vi "Package Must Exist.vi"(8 "error in (no error)":errorcluster, 11 "UpdateAction in":refnum<class "UpdateAction.lvclass">) -> (0 "error out":errorcluster, 2 "Pkg Must Exist":bool, 3 "UpdateAction out":refnum<class "UpdateAction.lvclass">)   [LabVIEW 2020, in "GPackTools.lvlib" / "UpdateAction.lvclass"]
uses:
  UpdateAction.lvclass
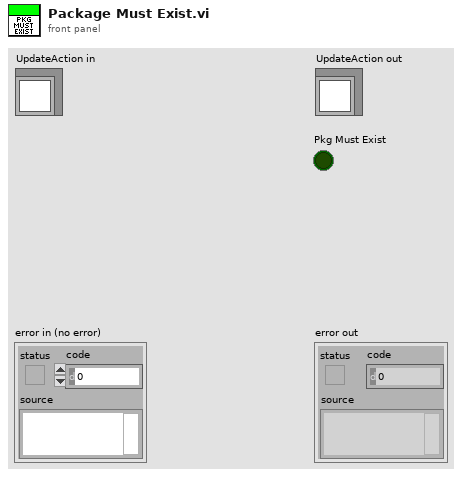
[diagram p1: front panel]
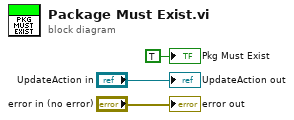
[diagram p0: block diagram]
diagram:
  "error out" <- "error in (no error)"
  "UpdateAction out" <- "UpdateAction in"
  "Pkg Must Exist" <- TRUE ("Pkg Must Exist")
